vi "ProcessMeaSplit.vi"(8 "error in (no error)":errorcluster, 10 "Data In":waveform(dbl)[](array[waveform]) caption="data", 11 "DAQList in":refnum<class "DAQList.lvclass">) -> (0 "error out":errorcluster, 2 "Data Out":waveform(dbl)[](array[waveform]) caption="data", 3 "DAQList out":refnum<class "DAQList.lvclass">)   [LabVIEW 2019, in "XCP_DaqDtoId.lvlib" / "DAQList.lvclass"]
uses:
  DAQList.lvclass
  DAQList.lvclass/DAQList.ctl
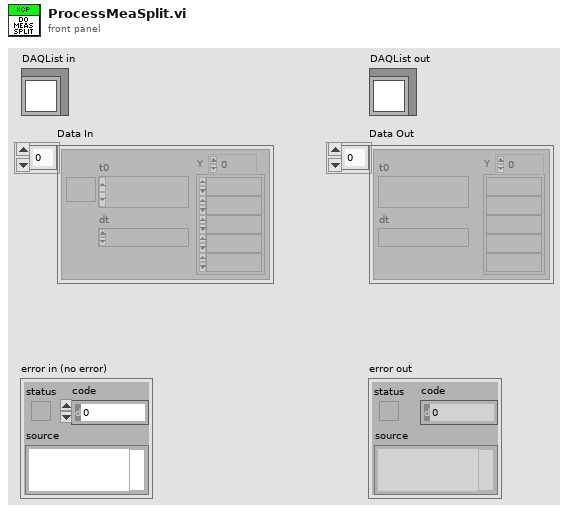
[diagram p1: front panel]
types:
  T1 = typedef "XCP_DaqDtoId.lvlib/DAQList.lvclass/MeaSplitInfo2.ctl" = cluster{"First Signal Index":i32, "Data Type":u32, "Byte Order":u32, "Scaling Offset":dbl, "Scaling Factor":dbl, "Numbers of Bytes":i32[]}
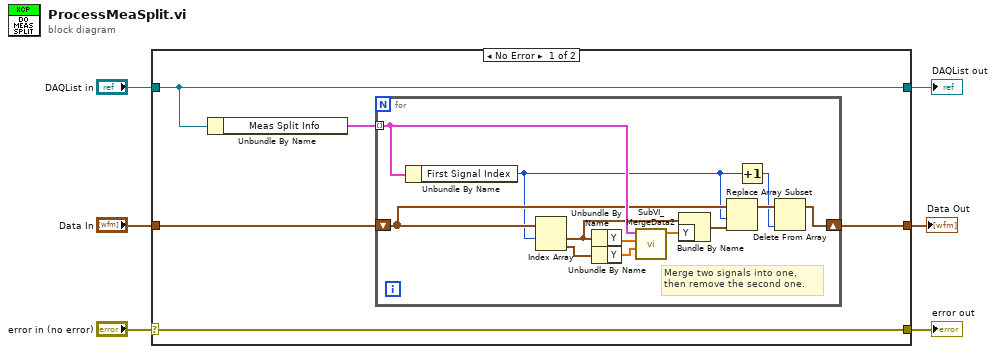
[diagram p0: block diagram]
diagram:
  n1 = case shown="No Error" "error in (no error)" {
    selector: "error in (no error)" -> [w11 w26]
    tunnel: [w11 w26] -> w5
    tunnel: [w10 w25] -> w3
    tunnel: "DAQList in" -> [w10 w25]
    tunnel: "Data In" -> [w8 w24]
    tunnel: [w7 w24] -> w1
    frame No Error {
      n2 = Unbundle By Name(w10) -> ("Meas Split Info"=w9:T1[])
      n3 = for {
        tunnel: w9 -> [w22] mode=indexing
        shift-right: [w12] -> w7
        shift-left: w8 -> [w17]
        # "Merge two signals into one, then remove the second one."
        n4 = Unbundle By Name(w22) -> ("First Signal Index"=w14:i32)
        n5 = Index Array(array=w17, index #1=w14) -> (element #1=w19:waveform(dbl), element #2=w23:waveform(dbl))  [unwired: 1 in]
        n6 = Unbundle By Name(w19) -> ("Y"=w21:dbl[])
        n7 = Unbundle By Name(w23) -> ("Y"=w20:dbl[])
        n8 = call "SubVI_MergeData2.vi"("Data Part 2"=w20, "Data Part 1"=w21, "Meas Split Info"=w22) -> ("Merged Data"=w18:dbl[])  [unwired: 8 in]
        n9 = Bundle By Name(cluster=w19, "Y"=w18) -> (w16:waveform(dbl))
        n10 = Replace Array Subset(array=w17, new element=w16, index=w14) -> (w15:waveform(dbl)[])
        n11 = Increment(x=w14) -> (x+1=w13:i32)
        n12 = Delete From Array(array=w15, index=w13) -> (array with subset deleted=w12:waveform(dbl)[])  [unwired: 1 in, 1 out]
      }
    }
    frame Error {
    }
  }
  "error out" <- w5
  "DAQList out" <- w3
  "Data Out" <- w1
